vi "Kalman filter - K array (SubVI).vi"(1 "R_measure":dbl, 2 "P Array in":dbl[][](array[numeric]), 3 "K Array in":dbl[](array[numeric])) -> (0 "K Array out":dbl[](array[numeric]))   [LabVIEW 2013]
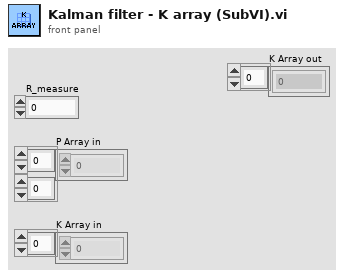
[diagram p1: front panel]
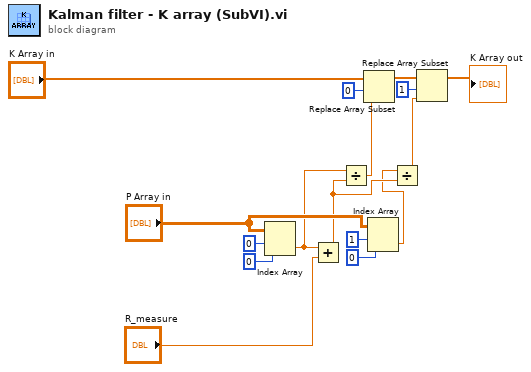
[diagram p0: block diagram]
diagram:
  n1 = Index Array(array="P Array in", index (row)=0, index (col)=0 ("disabled index (col)")) -> (element=w7:dbl)
  n2 = Add(x=w7, y="R_measure") -> (x+y=w14:dbl)
  n3 = Divide(x=w7, y=w14) -> (x/y=w8:dbl)
  n4 = Replace Array Subset(array="K Array in", new element=w8, index=0) -> (w9:dbl[])
  n5 = Index Array(array="P Array in", index (row)=1, index (col)=0) -> (element=w13:dbl)
  n6 = Divide(x=w13, y=w14) -> (x/y=w15:dbl)
  n7 = Replace Array Subset(array=w9, new element=w15, index=1) -> (→"K Array out":dbl[])
